vi "octave_demo.vi"() -> ()   [LabVIEW 2011]
doc: "Simple Octave interface demo."
uses:
  <vilib>/event_ctls.llb/eventvkey.ctl
panel:
  in  "use stderr":bool
  in  "read buffer size":i32=8192
  in  "recieve interval [ms]":i32=200
  out "running":bool
  in  "timeout [ms]":i32=2000
  in  "command":string
  out "response":string
  out "version":string
  in  "btn cmd":bool
  out "exit code":i32
  in  "open timeout [ms]":i32=30000
  in  "folder":path=path "C:/Octave/Octave3.6.4_gcc4.6.2/bin"
  in  "command line":string="octave.exe -q"
  out "error out":errorcluster
  in  "btn exit":bool
  in  "btn close":bool
  in  "btn open":bool
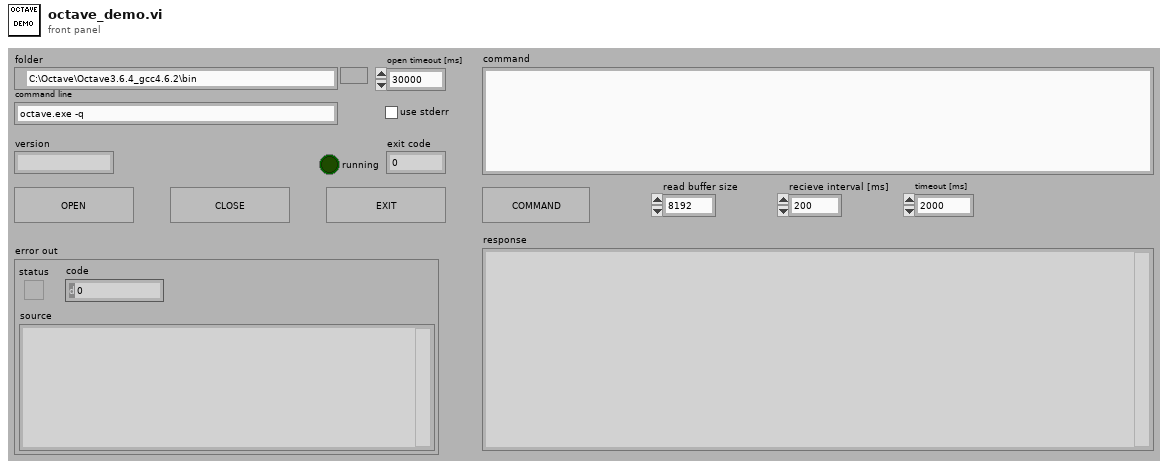
[diagram p1: front panel]
types:
  T1 = typedef "eventvkey.ctl" = enum16{"ASCII", "Enter", "Return", "Shift", "Ctrl", "Alt", "Cmd", "Opt", "Caps", "NumLock", "Clear", "Break", "Up", "Down", "Left", "Right", "Insert", "Delete", "Home", "End", "PageUp", "PageDown", "Escape", "Help", "Pause", "ScrollLock", "F1", "F2", "F3", "F4", "F5", "F6", "F7", "F8", "F9", "F10", "F11", "F12", "F13", "F14", "F15", "F16", "F17", "F18", "F19", "F20", "F21", "F22", "F23", "F24", "Play", "VolumeUp", "VolumeDown", "Mute", "Two Byte Char"}
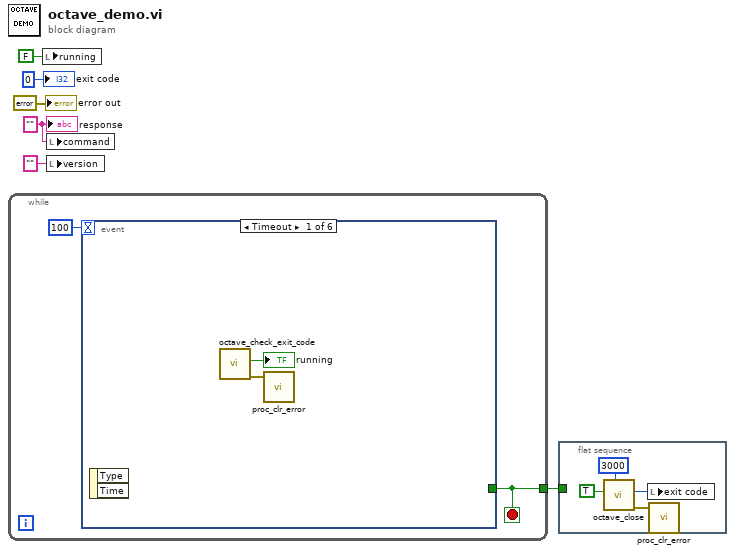
[diagram p0: block diagram]
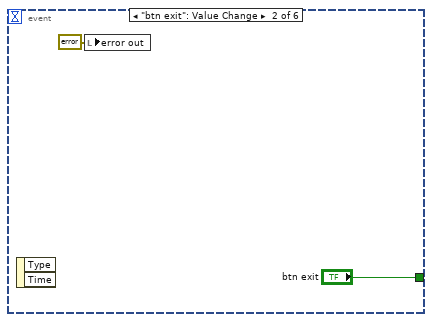
[diagram p2: hidden frame]
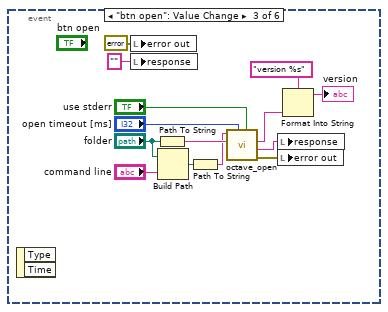
[diagram p3: hidden frame]
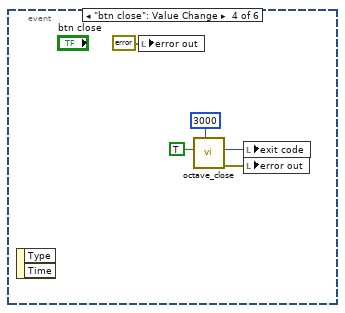
[diagram p4: hidden frame]
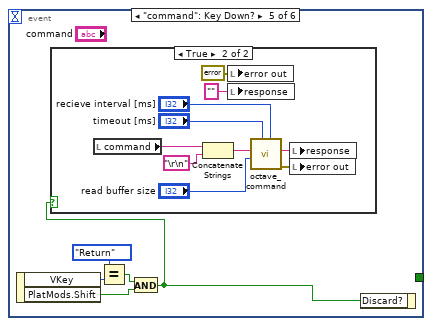
[diagram p5: hidden frame]
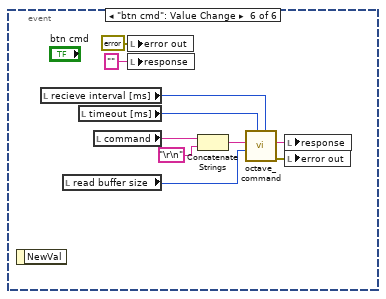
[diagram p7: hidden frame]
diagram:
  w3 = "" ("response")
  n1 = while {
    tunnel: [w8] -> w4
    stop <- w8 stop-if-true
    n2 = event shown="[0] Timeout" {
      selector: _ -> [_ _ _ _ _ _]
      dyn-events: _ -> [_ _ _ _ _ _]
      timeout: 100 -> [_ _ _ _ _ _]
      tunnel: [_ "btn exit" _ _ _ _] -> w8
      event Timeout {
        n3 = event-data() -> ()  [unwired: 1 in, 2 out]
        n4 = call "octave_check_exit_code.vi"() -> ("error out"=w10:errorcluster, "running"=→"running":bool)  [unwired: 7 in, 3 out]
        n5 = call "proc_clr_error.vi"("error in (no error)"=w10) -> ()  [unwired: 4 in, 1 out]
      }
      event "btn exit": Value Change {
        n6 = event-data() -> ()  [unwired: 1 in, 2 out]
        n7 = local write "error out"(errorcluster {"status"=FALSE, "code"=0, "source"=""} ("error out")) -> ()
      }
      event "btn open": Value Change {
        n8 = event-data() -> ()  [unwired: 1 in, 2 out]
        n9 = local write "error out"(errorcluster {"status"=FALSE, "code"=0, "source"=""} ("error out")) -> ()
        n10 = local write "response"("" ("command")) -> ()
        n11 = Path To String(path="folder") -> (string=w18:string)
        n12 = Build Path(base path="folder", name or relative path="command line") -> (appended path=w17:path)
        n13 = Path To String(path=w17) -> (string=w16:string)
        n14 = call "octave_open.vi"("use stderr"="use stderr", "timeout [ms]"="open timeout [ms]", "folder"=w18, "command"=w16) -> ("error out"=w26:errorcluster, "initial garbage"=w14:string, "version string"=w13:string)  [unwired: 4 in, 1 out]
        n15 = local write "response"(w14) -> ()
        n16 = local write "error out"(w26) -> ()
        n17 = Format Into String(format string="version %s", w13) -> (resulting string=→"version":string)  [unwired: 2 in, 1 out]
      }
      event "btn close": Value Change {
        n18 = event-data() -> ()  [unwired: 1 in, 2 out]
        n19 = local write "error out"(errorcluster {"status"=FALSE, "code"=0, "source"=""} ("error out")) -> ()
        n20 = call "octave_close.vi"("timeout [ms]"=3000, "try kill if error"=TRUE ("terminate if error")) -> ("error out"=w30:errorcluster, "exit code"=w27:i32)  [unwired: 6 in, 2 out]
        n21 = local write "exit code"(w27) -> ()
        n22 = local write "error out"(w30) -> ()
      }
      event "command": Key Down? {
        n23 = event-data() -> ("VKey"=w36:T1, "PlatMods.Shift"=w34:bool)  [unwired: 1 in]
        n24 = Equal?(x=eventvkey."Return", y=w36) -> (x = y?=w33:bool)
        n25 = And(x=w33, y=w34) -> (x .and. y?=w32:bool)
        n26 = case shown="True" w32 {
          frame False {
          }
          frame True {
            n27 = local read "command"() -> (w37:string)
            n28 = Concatenate Strings(w37, "\r\n") -> (w39:string)
            n29 = local write "error out"(errorcluster {"status"=FALSE, "code"=0, "source"=""} ("error out")) -> ()
            n30 = local write "response"("" ("response")) -> ()
            n31 = call "octave_command.vi"("recieve interval [ms]"="recieve interval [ms]", "timeout [ms]"="timeout [ms]", "read buffer size (4096)"="read buffer size", "write buffer"=w39) -> ("error out"=w45:errorcluster, "read buffer"=w40:string)  [unwired: 3 in, 3 out]
            n32 = local write "response"(w40) -> ()
            n33 = local write "error out"(w45) -> ()
          }
        }
        n34 = event-data("Discard?"=w32) -> ()  [unwired: 1 in, 1 out]
      }
      event "btn cmd": Value Change {
        n35 = event-data() -> ()  [unwired: 1 in, 1 out]
        n36 = local read "recieve interval [ms]"() -> (w50:i32)
        n37 = local read "read buffer size"() -> (w48:i32)
        n38 = local read "timeout [ms]"() -> (w49:i32)
        n39 = local read "command"() -> (w47:string)
        n40 = local write "error out"(errorcluster {"status"=FALSE, "code"=0, "source"=""} ("error out")) -> ()
        n41 = local write "response"("" ("response")) -> ()
        n42 = Concatenate Strings(w47, "\r\n") -> (w51:string)
        n43 = call "octave_command.vi"("recieve interval [ms]"=w50, "timeout [ms]"=w49, "read buffer size (4096)"=w48, "write buffer"=w51) -> ("error out"=w55:errorcluster, "read buffer"=w52:string)  [unwired: 3 in, 3 out]
        n44 = local write "response"(w52) -> ()
        n45 = local write "error out"(w55) -> ()
      }
    }
  }
  n46 = local write "running"(FALSE ("running")) -> ()
  n47 = local write "command"(w3) -> ()
  n48 = local write "version"("" ("version")) -> ()
  n49 = flat-sequence {
    tunnel: w4 -> [_]
    frame #0 {
      n50 = call "octave_close.vi"("timeout [ms]"=3000, "try kill if error"=TRUE ("terminate if error")) -> ("error out"=w60:errorcluster, "exit code"=w57:i32)  [unwired: 6 in, 2 out]
      n51 = local write "exit code"(w57) -> ()
      n52 = call "proc_clr_error.vi"("error in (no error)"=w60) -> ()  [unwired: 4 in, 1 out]
    }
  }
  "error out" <- errorcluster {"status"=FALSE, "code"=0, "source"=""} ("error out")
  "response" <- w3
  "exit code" <- 0 ("exit code")
